vi "openFpga.vi"(8 "error in (no error)":errorcluster, 11 "FpgaRunner in":refnum<class "FpgaRunner.lvclass">) -> (0 "error out":errorcluster, 3 "FpgaRunner out":refnum<class "FpgaRunner.lvclass">)   [LabVIEW 2020, in "FpgaRunner.lvclass"]
uses:
  FpgaRunner.lvclass
  <vilib>/rvi/interface/nirviOpenFPGA/nirviOpenFPGA.xnode
  fpga/fpga.sandbox.ip.vi
  <vilib>/rvi/interface/nirviUpCast/nirviUpCast.xnode
  FPGA Bitfiles/market.data.poc_FPGATarget_poc.ip.kria_VbtSJiBgbQ0.lvbitx
  fpga/poc.ip.kria.vi
  <vilib>/FPGAPlugInAG/USRP-X410/niLvFpga_Open_USRP-X410.vi
  <vilib>/rvi/interface/common/dynamic/niFpgaDynamicAddResources.vi
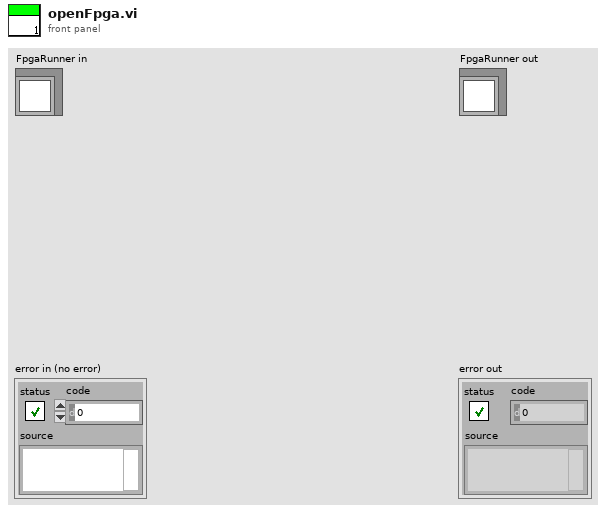
[diagram p1: front panel]
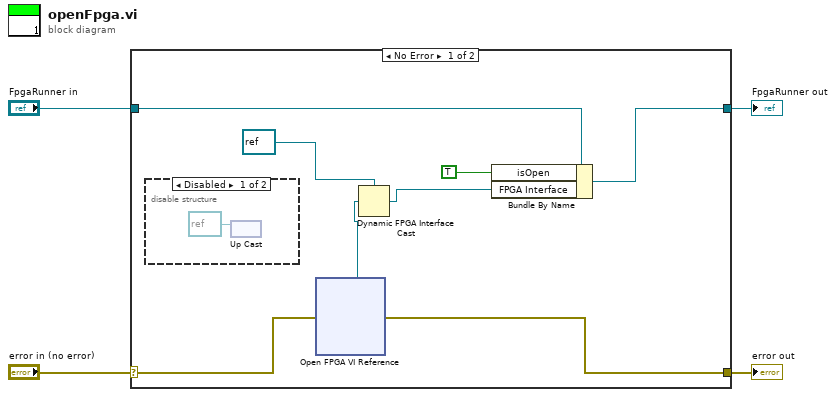
[diagram p0: block diagram]
diagram:
  n1 = case shown="No Error" "error in (no error)" {
    selector: "error in (no error)" -> [w12 w22]
    tunnel: [w11 w22] -> w3
    tunnel: [w8 w21] -> w1
    tunnel: "FpgaRunner in" -> [w10 w21]
    frame No Error {
      n2 = disable-structure shown="Disabled" {
        frame Disabled {
          n3 = xnode "Up Cast"("FPGA VI Reference In"=refnum<k20> refnum) -> ()  [unwired: 1 in, 2 out]
        }
        frame Enabled {
        }
      }
      n4 = xnode "Open FPGA VI Reference"("error in"=w12) -> ("FPGA VI Reference Out"=w5:refnum<k20>, "error out"=w11:errorcluster)  [unwired: 1 in]
      n5 = Dynamic FPGA Interface Cast(Session In=refnum<k20> refnum ("FPGA Interface"), Type=w5) -> (Session Out=w6:refnum<k20>)
      n6 = Bundle By Name(cluster=w10, "isOpen"=TRUE, "FPGA Interface"=w6) -> (w8:refnum<class "FpgaRunner.lvclass">)
    }
    frame Error {
    }
  }
  "error out" <- w3
  "FpgaRunner out" <- w1
